vi "FS Operation Plane.vi"(6 "Plane #":i32=1, 9 "Plane Specs":T1={"Origin"={"X"=0.0, "Y"=0.0, "Z"=6.0}, "Normal"={"X"=0.0, "Y"=0.0, "Z"=1.0}, "X Direction"={"X"=1.0, "Y"=0.0, "Z"=0.0}, "Size"={"Width"=6.0, "Height"=6.0}}, 11 "Feature In":string="FeatureScript 1247;\nimport(path : \"onshape/std/geometry.fs\", version : \"1247.0\");\n\nannotation { \"Feature Type Name\" : \"LabVIEW Feature\" }\nexport const myFeature = defineFeature(function(context is Context, id is Id, definition is map)\n    precondition\n    {\n        // Define the parameters of the feature type\n    }\n    {\n        // Define the function's action\n    });") -> (3 "Feature Out":string="FeatureScript 1247;\nimport(path : \"onshape/std/geometry.fs\", version : \"1247.0\");\n\nannotation { \"Feature Type Name\" : \"LVFeat1\" }\nexport const myFeature = defineFeature(function(context is Context, id is Id, definition is map)\n    precondition\n    {\n        // Define the parameters of the feature type\n    }\n    {\n        // Define the function's action\n\nvar sketch1 = newSketch(context, id + \"sketch1\", {\n                \"sketchPlane\" : qCreatedBy(makeId(\"Top\"), EntityType.FACE)\n        });\n        // Create sketch entities here\n        skRectangle(sketch1, \"rectangle1\", {\n                \"firstCorner\" : vector(0, 0) * inch,\n                \"secondCorner\" : vector(3, 4) * inch\n        });\n        \n        skSolve(sketch1);\n    });")   [LabVIEW 2019]
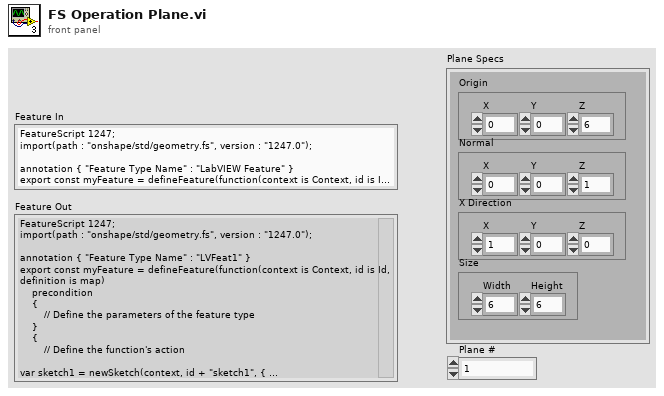
[diagram p1: front panel]
types:
  T1 = cluster{"Origin":cluster{"X":dbl, "Y":dbl, "Z":dbl}, "Normal":cluster{"X":dbl, "Y":dbl, "Z":dbl}, "X Direction":cluster{"X":dbl, "Y":dbl, "Z":dbl}, "Size":cluster{"Width":dbl, "Height":dbl}}
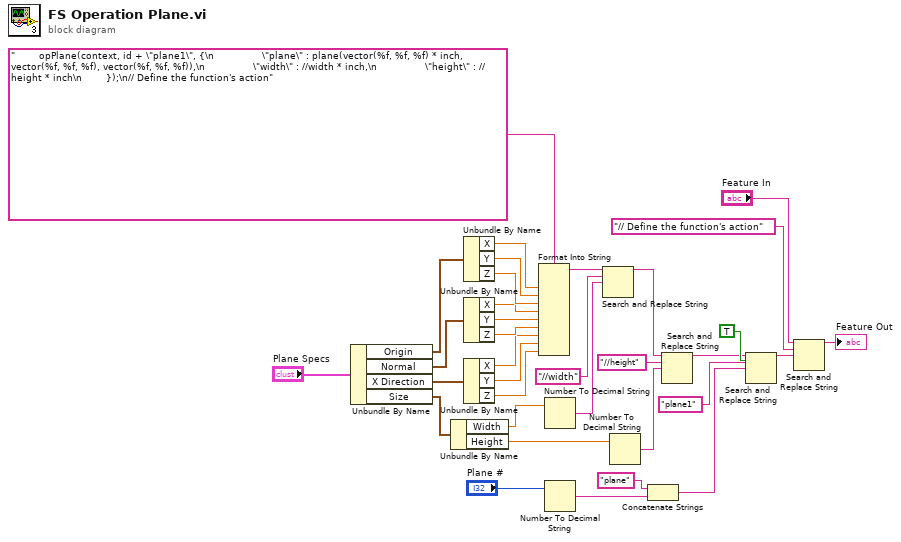
[diagram p0: block diagram]
diagram:
  n1 = Unbundle By Name("Plane Specs") -> ("Origin"=w21:cluster{"X":dbl, "Y":dbl, "Z":dbl}, "Normal"=w20:cluster{"X":dbl, "Y":dbl, "Z":dbl}, "X Direction"=w19:cluster{"X":dbl, "Y":dbl, "Z":dbl}, "Size"=w18:cluster{"Width":dbl, "Height":dbl})
  n2 = Unbundle By Name(w18) -> ("Width"=w17:dbl, "Height"=w12:dbl)
  n3 = Unbundle By Name(w21) -> ("X"=w11:dbl, "Y"=w10:dbl, "Z"=w9:dbl)
  n4 = Unbundle By Name(w20) -> ("X"=w8:dbl, "Y"=w7:dbl, "Z"=w6:dbl)
  n5 = Unbundle By Name(w19) -> ("X"=w5:dbl, "Y"=w4:dbl, "Z"=w3:dbl)
  n6 = Format Into String(format string="        opPlane(context, id + \"plane1\", {\n                \"plane\" : plane(vector(%f, %f, %f) * inch, vector(%f, %f, %f), vector(%f, %f, %f)),\n                \"width\" : //width * inch,\n                \"height\" : //height * inch\n        });\n// Define the function's action" ("search string"), w11, w10, w9, w8, w7, w6, w5, w4, w3) -> (resulting string=w1:string)  [unwired: 2 in, 1 out]
  n7 = Number To Decimal String(number=w17) -> (decimal integer string=w24:string)  [unwired: 1 in]
  n8 = Number To Decimal String(number="Plane #") -> (decimal integer string=w26:string)  [unwired: 1 in]
  n9 = Search and Replace String(input string=w1, search string="//width", replace string=w24) -> (result string=w14:string)  [unwired: 5 in, 3 out]
  n10 = Number To Decimal String(number=w12) -> (decimal integer string=w15:string)  [unwired: 1 in]
  n11 = Concatenate Strings("plane" ("regular expression"), w26) -> (w30:string)
  n12 = Search and Replace String(input string=w14, search string="//height", replace string=w15) -> (result string=w13:string)  [unwired: 5 in, 3 out]
  n13 = Search and Replace String(replace all?=TRUE ("replace all? (F)"), input string=w13, search string="plane1" ("regular expression"), replace string=w30) -> (result string=w25:string)  [unwired: 4 in, 3 out]
  n14 = Search and Replace String(input string="Feature In", search string="// Define the function's action", replace string=w25) -> (result string=→"Feature Out":string)  [unwired: 5 in, 3 out]
